vi "Pre Launch Init.vi"(11 "Logging in":refnum<class "Logging.lvclass">) -> (0 "error out":errorcluster, 3 "Logging out":refnum<class "Logging.lvclass">)   [LabVIEW 2020, in "Logging.lvlib" / "Logging.lvclass"]
doc: "Initializes the panel actor. Creates the Panel Helper.\n\n----\nPlease see the following web address for additional documentation and tutorial information:\nhttp://www.mooregoodideas.com/mgi-panel-manager/\n\nAuthor: Derek Trepanier\n\nCopyright (c) 2018, Moore Good Ideas, Inc.\n\nAll rights reserved.\n\nRedistribution and use in source and binary forms, with or without modification, are permitted provided that the following conditions are met:\n\n * Redistributions of source code must retain the above copyright notice, this list of conditions and the following disclaimer.\n * Redistributions in binary form must reproduce the above copyright notice, this list of conditions and the following disclaimer in the documentation and/or other materials provided with the distribution.\n * Neither the name of Moore Good Ideas, Inc. nor the names of its contributors may be used to endorse or promote products derived from this software without specific prior written permission.\n\nTHIS SOFTWARE IS PROVIDED BY THE COPYRIGHT HOLDERS AND CONTRIBUTORS \"AS IS\" AND ANY EXPRESS OR IMPLIED WARRANTIES, INCLUDING, BUT NOT LIMITED TO, THE IMPLIED WARRANTIES OF MERCHANTABILITY AND FITNESS FOR A PARTICULAR PURPOSE ARE DISCLAIMED. IN NO EVENT SHALL THE COPYRIGHT OWNER OR CONTRIBUTORS BE LIABLE FOR ANY DIRECT, INDIRECT, INCIDENTAL, SPECIAL, EXEMPLARY, OR CONSEQUENTIAL DAMAGES (INCLUDING, BUT NOT LIMITED TO, PROCUREMENT OF SUBSTITUTE GOODS OR SERVICES; LOSS OF USE, DATA, OR PROFITS; OR BUSINESS INTERRUPTION) HOWEVER CAUSED AND ON ANY THEORY OF LIABILITY, WHETHER IN CONTRACT, STRICT LIABILITY, OR TORT (INCLUDING NEGLIGENCE OR OTHERWISE) ARISING IN ANY WAY OUT OF THE USE OF THIS SOFTWARE, EVEN IF ADVISED OF THE POSSIBILITY OF SUCH DAMAGE."
uses:
  Logging.lvclass
  Logging.lvclass/Logging.ctl
  <vilib>/MGI/Panel Manager/Panel Actor/Panel Actor/Panel Actor.lvclass
  <vilib>/Utility/file.llb/Read Delimited Spreadsheet (DBL).vi
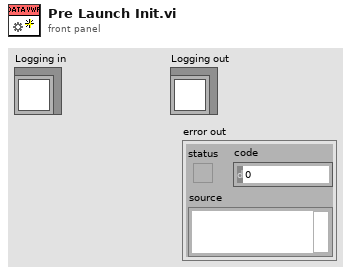
[diagram p1: front panel]
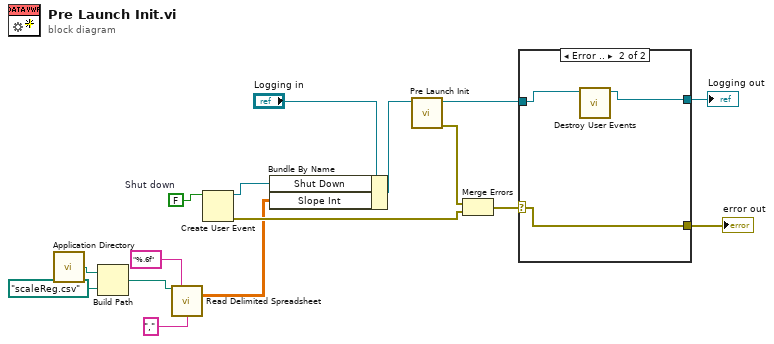
[diagram p0: block diagram]
diagram:
  w14 = FALSE  # Shut down
  n1 = call <vilib>:"Application Directory.vi"() -> ("Application Directory"=w6:path)
  n2 = Build Path(base path=w6, name or relative path=path "scaleReg.csv") -> (appended path=w4:path)
  n3 = call-poly <vilib>:"Read Delimited Spreadsheet.vi"("file path (dialog if empty)"=w4, "format (%.3f)"="%.6f", "delimiter (\\t)"="," ("delimiter (\\t)")) -> ("all rows"=w1:dbl[][])  [unwired: 7 in, 5 out]
  n4 = Create User Event(user event datatype=w14) -> (user event=w13:refnum<user-event>, error out=w11:errorcluster)  [unwired: 1 in]
  n5 = Bundle By Name(cluster="Logging in", "Shut Down"=w13, "Slope Int"=w1) -> (w15:refnum<class "Logging.lvclass">)
  n6 = call-parent "Pre Launch Init.vi"("Panel Actor in"=w15) -> ("error out"=w12:errorcluster, "Panel Actor out"=w9:refnum<class "Logging.lvclass">)  [unwired: 9 in]
  n7 = Merge Errors(w12, w11) -> (w10:errorcluster)
  n8 = case shown="Error .." w10 {
    selector: w10 -> [w17 w21]
    tunnel: w9 -> [w18 w20]
    tunnel: [w18 w19] -> w8
    tunnel: [w17 w21] -> w7
    frame No Error {
    }
    frame Error {
      n9 = call "Destroy User Events.vi"("Logging in"=w20) -> ("Logging out"=w19:refnum<class "Logging.lvclass">)  [unwired: 10 in]
    }
  }
  "error out" <- w7
  "Logging out" <- w8
